vi "S4GUI_003.vi"(7 "Tab ObsEng":enum32{"Obs", "CCD modes", "Guider", "Eng"}(tab)) -> ()   [LabVIEW 2018] (continued)
                n3340 = call-dynamic "Read Interface.vi"("error in (no error)"=w7310, "Channel in"=w7313) -> ("error out"=w7327:errorcluster, "Interface.lvclass"=w7328:refnum<class "Interface.lvclass">, "Channel out"=w7345:refnum<class "Channel.lvclass">)  [unwired: 7 in]
                n3341 = call-dynamic "Write Suffix.vi"("error in (no error)"=w7327, "Suffix"=w7335, "Interface in"=w7328) -> ("error out"=w7352:errorcluster, "Interface out"=w7344:refnum<class "Interface.lvclass">)  [unwired: 7 in]
                n3342 = call-dynamic "Write ObsType.vi"("error in (no error)"=w7352, "ObsType"=w7333, "Interface in"=w7344) -> ("error out"=w7351:errorcluster, "Interface out"=w7343:refnum<class "Interface.lvclass">)  [unwired: 7 in]
                n3343 = call-dynamic "Write Object.vi"("error in (no error)"=w7351, "Object"=w7332, "Interface in"=w7343) -> ("error out"=w7350:errorcluster, "Interface out"=w7342:refnum<class "Interface.lvclass">)  [unwired: 7 in]
                n3344 = call-dynamic "Write Comments.vi"("error in (no error)"=w7350, "Comments"=w7334, "Interface in"=w7342) -> ("error out"=w7330:errorcluster, "Interface out"=w7329:refnum<class "Interface.lvclass">)  [unwired: 7 in]
                n3345 = call-dynamic "Write Observer.vi"("error in (no error)"=w7330, "Observer"=w7331, "Interface in"=w7329) -> ("error out"=w7325:errorcluster, "Interface out"=w7326:refnum<class "Interface.lvclass">)  [unwired: 7 in]
                n3346 = call-dynamic "Write Interface.vi"("error in (no error)"=w7325, "Interface.lvclass"=w7326, "Channel in"=w7345) -> ("error out"=w7321:errorcluster, "Channel out"=w7324:refnum<class "Channel.lvclass">)  [unwired: 7 in]
                n3347 = call-dynamic "Read State Machine.vi"("error in (no error)"=w7321, "Device in"=w7324) -> ("error out"=w7320:errorcluster, "State Machine.lvclass"=w7318:refnum<class "State Machine.lvclass">, "Device out"=w7323:refnum<class "Channel.lvclass">)  [unwired: 7 in]
                n3348 = call "Next State.vi"("error in (no error)"=w7320, "New_State"=12, "State Machine in"=w7318) -> ("error out"=w7319:errorcluster, "State Machine out"=w7317:refnum<class "State Machine.lvclass">)  [unwired: 7 in]
                n3349 = call-dynamic "Write State Machine.vi"("error in (no error)"=w7319, "State Machine.lvclass"=w7317, "Device in"=w7323) -> ("error out"=w7316:errorcluster, "Device out"=w7322:refnum<class "Channel.lvclass">)  [unwired: 7 in]
                n3350 = call-dynamic "Write Channel.vi"("error in (no error)"=w7316, "Channel.lvclass"=w7322, "Acquisition in"=w7340) -> ("error out"=w7338:errorcluster, "Acquisition out"=w7339:refnum<class "Acquisition.lvclass">)  [unwired: 7 in]
                n3351 = call-dynamic "Write AcquisitionA.vi"("error in (no error)"=w7338, "Acquisition.lvclass"=w7339, "S4ACS_GUI in"=w7341) -> ("error out"=w7336:errorcluster, "S4ACS_GUI out"=w7337:refnum<class "S4GUI.lvclass">)  [unwired: 7 in]
              }
              frame #1 {
                # "object"
                # "suffix"
                # "obsType"
                n3352 = call "Read AcquisitionB.vi"("error in (no error)"=w7394, "S4ACS_GUI in"=w7395) -> ("error out"=w7380:errorcluster, "Acquisition.lvclass"=w7381:refnum<class "Acquisition.lvclass">, "S4ACS_GUI out"=w7386:refnum<class "S4GUI.lvclass">)  [unwired: 7 in]
                n3353 = call-dynamic "Read Channel.vi"("error in (no error)"=w7380, "Acquisition in"=w7381) -> ("error out"=w7354:errorcluster, "Channel.lvclass"=w7356:refnum<class "Channel.lvclass">, "Acquisition out"=w7387:refnum<class "Acquisition.lvclass">)  [unwired: 7 in]
                n3354 = local read "Filter2"() -> (w7357:u8)
                n3355 = call-dynamic "Write Filter.vi"("error in (no error)"=w7354, "Filter"=w7357, "Channel in"=w7356) -> ("error out"=w7353:errorcluster, "Channel out"=w7355:refnum<class "Channel.lvclass">)  [unwired: 7 in]
                n3356 = call-dynamic "Read Interface.vi"("error in (no error)"=w7353, "Channel in"=w7355) -> ("error out"=w7368:errorcluster, "Interface.lvclass"=w7369:refnum<class "Interface.lvclass">, "Channel out"=w7382:refnum<class "Channel.lvclass">)  [unwired: 7 in]
                n3357 = call-dynamic "Write Suffix.vi"("error in (no error)"=w7368, "Suffix"=w7391, "Interface in"=w7369) -> ("error out"=w7377:errorcluster, "Interface out"=w7383:refnum<class "Interface.lvclass">)  [unwired: 7 in]
                n3358 = call-dynamic "Write ObsType.vi"("error in (no error)"=w7377, "ObsType"=w7376, "Interface in"=w7383) -> ("error out"=w7378:errorcluster, "Interface out"=w7384:refnum<class "Interface.lvclass">)  [unwired: 7 in]
                n3359 = call-dynamic "Write Object.vi"("error in (no error)"=w7378, "Object"=w7375, "Interface in"=w7384) -> ("error out"=w7379:errorcluster, "Interface out"=w7385:refnum<class "Interface.lvclass">)  [unwired: 7 in]
                n3360 = call-dynamic "Write Comments.vi"("error in (no error)"=w7379, "Comments"=w7390, "Interface in"=w7385) -> ("error out"=w7371:errorcluster, "Interface out"=w7370:refnum<class "Interface.lvclass">)  [unwired: 7 in]
                n3361 = call-dynamic "Write Observer.vi"("error in (no error)"=w7371, "Observer"=w7374, "Interface in"=w7370) -> ("error out"=w7372:errorcluster, "Interface out"=w7373:refnum<class "Interface.lvclass">)  [unwired: 7 in]
                n3362 = call-dynamic "Write Interface.vi"("error in (no error)"=w7372, "Interface.lvclass"=w7373, "Channel in"=w7382) -> ("error out"=w7361:errorcluster, "Channel out"=w7362:refnum<class "Channel.lvclass">)  [unwired: 7 in]
                n3363 = call-dynamic "Read State Machine.vi"("error in (no error)"=w7361, "Device in"=w7362) -> ("error out"=w7367:errorcluster, "State Machine.lvclass"=w7365:refnum<class "State Machine.lvclass">, "Device out"=w7360:refnum<class "Channel.lvclass">)  [unwired: 7 in]
                n3364 = call "Next State.vi"("error in (no error)"=w7367, "New_State"=12, "State Machine in"=w7365) -> ("error out"=w7366:errorcluster, "State Machine out"=w7364:refnum<class "State Machine.lvclass">)  [unwired: 7 in]
                n3365 = call-dynamic "Write State Machine.vi"("error in (no error)"=w7366, "State Machine.lvclass"=w7364, "Device in"=w7360) -> ("error out"=w7358:errorcluster, "Device out"=w7359:refnum<class "Channel.lvclass">)  [unwired: 7 in]
                n3366 = call-dynamic "Write Channel.vi"("error in (no error)"=w7358, "Channel.lvclass"=w7359, "Acquisition in"=w7387) -> ("error out"=w7389:errorcluster, "Acquisition out"=w7388:refnum<class "Acquisition.lvclass">)  [unwired: 7 in]
                n3367 = call "Write AcquisitionB.vi"("error in (no error)"=w7389, "Acquisition.lvclass"=w7388, "S4ACS_GUI in"=w7386) -> ("error out"=w7392:errorcluster, "S4ACS_GUI out"=w7393:refnum<class "S4GUI.lvclass">)  [unwired: 7 in]
              }
              frame #2 {
                # "object"
                # "suffix"
                # "obsType"
                n3368 = call-dynamic "Read AcquisitionC.vi"("error in (no error)"=w7437, "S4ACS_GUI in"=w7438) -> ("error out"=w7430:errorcluster, "Acquisition.lvclass"=w7429:refnum<class "Acquisition.lvclass">, "S4ACS_GUI out"=w7424:refnum<class "S4GUI.lvclass">)  [unwired: 7 in]
                n3369 = call-dynamic "Read Channel.vi"("error in (no error)"=w7430, "Acquisition in"=w7429) -> ("error out"=w7397:errorcluster, "Channel.lvclass"=w7399:refnum<class "Channel.lvclass">, "Acquisition out"=w7423:refnum<class "Acquisition.lvclass">)  [unwired: 7 in]
                n3370 = local read "Filter3"() -> (w7400:u8)
                n3371 = call-dynamic "Write Filter.vi"("error in (no error)"=w7397, "Filter"=w7400, "Channel in"=w7399) -> ("error out"=w7396:errorcluster, "Channel out"=w7398:refnum<class "Channel.lvclass">)  [unwired: 7 in]
                n3372 = call-dynamic "Read Interface.vi"("error in (no error)"=w7396, "Channel in"=w7398) -> ("error out"=w7415:errorcluster, "Interface.lvclass"=w7416:refnum<class "Interface.lvclass">, "Channel out"=w7428:refnum<class "Channel.lvclass">)  [unwired: 7 in]
                n3373 = call-dynamic "Write Suffix.vi"("error in (no error)"=w7415, "Suffix"=w7434, "Interface in"=w7416) -> ("error out"=w7433:errorcluster, "Interface out"=w7427:refnum<class "Interface.lvclass">)  [unwired: 7 in]
                n3374 = call-dynamic "Write ObsType.vi"("error in (no error)"=w7433, "ObsType"=w7419, "Interface in"=w7427) -> ("error out"=w7432:errorcluster, "Interface out"=w7426:refnum<class "Interface.lvclass">)  [unwired: 7 in]
                n3375 = call-dynamic "Write Object.vi"("error in (no error)"=w7432, "Object"=w7418, "Interface in"=w7426) -> ("error out"=w7431:errorcluster, "Interface out"=w7425:refnum<class "Interface.lvclass">)  [unwired: 7 in]
                n3376 = call-dynamic "Write Comments.vi"("error in (no error)"=w7431, "Comments"=w7420, "Interface in"=w7425) -> ("error out"=w7412:errorcluster, "Interface out"=w7411:refnum<class "Interface.lvclass">)  [unwired: 7 in]
                n3377 = call-dynamic "Write Observer.vi"("error in (no error)"=w7412, "Observer"=w7417, "Interface in"=w7411) -> ("error out"=w7413:errorcluster, "Interface out"=w7414:refnum<class "Interface.lvclass">)  [unwired: 7 in]
                n3378 = call-dynamic "Write Interface.vi"("error in (no error)"=w7413, "Interface.lvclass"=w7414, "Channel in"=w7428) -> ("error out"=w7406:errorcluster, "Channel out"=w7407:refnum<class "Channel.lvclass">)  [unwired: 7 in]
                n3379 = call-dynamic "Read State Machine.vi"("error in (no error)"=w7406, "Device in"=w7407) -> ("error out"=w7410:errorcluster, "State Machine.lvclass"=w7403:refnum<class "State Machine.lvclass">, "Device out"=w7405:refnum<class "Channel.lvclass">)  [unwired: 7 in]
                n3380 = call "Next State.vi"("error in (no error)"=w7410, "New_State"=12, "State Machine in"=w7403) -> ("error out"=w7409:errorcluster, "State Machine out"=w7402:refnum<class "State Machine.lvclass">)  [unwired: 7 in]
                n3381 = call-dynamic "Write State Machine.vi"("error in (no error)"=w7409, "State Machine.lvclass"=w7402, "Device in"=w7405) -> ("error out"=w7401:errorcluster, "Device out"=w7404:refnum<class "Channel.lvclass">)  [unwired: 7 in]
                n3382 = call-dynamic "Write Channel.vi"("error in (no error)"=w7401, "Channel.lvclass"=w7404, "Acquisition in"=w7423) -> ("error out"=w7421:errorcluster, "Acquisition out"=w7422:refnum<class "Acquisition.lvclass">)  [unwired: 7 in]
                n3383 = call-dynamic "Write AcquisitionC.vi"("error in (no error)"=w7421, "Acquisition.lvclass"=w7422, "S4ACS_GUI in"=w7424) -> ("error out"=w7435:errorcluster, "S4ACS_GUI out"=w7436:refnum<class "S4GUI.lvclass">)  [unwired: 7 in]
              }
              frame #3 {
                # "object"
                # "suffix"
                # "obsType"
                n3384 = call-dynamic "Read AcquisitionD.vi"("error in (no error)"=w7480, "S4ACS_GUI in"=w7481) -> ("error out"=w7473:errorcluster, "Acquisition.lvclass"=w7472:refnum<class "Acquisition.lvclass">, "S4ACS_GUI out"=w7467:refnum<class "S4GUI.lvclass">)  [unwired: 7 in]
                n3385 = call-dynamic "Read Channel.vi"("error in (no error)"=w7473, "Acquisition in"=w7472) -> ("error out"=w7440:errorcluster, "Channel.lvclass"=w7442:refnum<class "Channel.lvclass">, "Acquisition out"=w7466:refnum<class "Acquisition.lvclass">)  [unwired: 7 in]
                n3386 = local read "Filter4"() -> (w7443:u8)
                n3387 = call-dynamic "Write Filter.vi"("error in (no error)"=w7440, "Filter"=w7443, "Channel in"=w7442) -> ("error out"=w7439:errorcluster, "Channel out"=w7441:refnum<class "Channel.lvclass">)  [unwired: 7 in]
                n3388 = call-dynamic "Read Interface.vi"("error in (no error)"=w7439, "Channel in"=w7441) -> ("error out"=w7458:errorcluster, "Interface.lvclass"=w7459:refnum<class "Interface.lvclass">, "Channel out"=w7471:refnum<class "Channel.lvclass">)  [unwired: 7 in]
                n3389 = call-dynamic "Write Suffix.vi"("error in (no error)"=w7458, "Suffix"=w7477, "Interface in"=w7459) -> ("error out"=w7476:errorcluster, "Interface out"=w7470:refnum<class "Interface.lvclass">)  [unwired: 7 in]
                n3390 = call-dynamic "Write ObsType.vi"("error in (no error)"=w7476, "ObsType"=w7462, "Interface in"=w7470) -> ("error out"=w7475:errorcluster, "Interface out"=w7469:refnum<class "Interface.lvclass">)  [unwired: 7 in]
                n3391 = call-dynamic "Write Object.vi"("error in (no error)"=w7475, "Object"=w7461, "Interface in"=w7469) -> ("error out"=w7474:errorcluster, "Interface out"=w7468:refnum<class "Interface.lvclass">)  [unwired: 7 in]
                n3392 = call-dynamic "Write Comments.vi"("error in (no error)"=w7474, "Comments"=w7463, "Interface in"=w7468) -> ("error out"=w7457:errorcluster, "Interface out"=w7456:refnum<class "Interface.lvclass">)  [unwired: 7 in]
                n3393 = call-dynamic "Write Observer.vi"("error in (no error)"=w7457, "Observer"=w7460, "Interface in"=w7456) -> ("error out"=w7452:errorcluster, "Interface out"=w7451:refnum<class "Interface.lvclass">)  [unwired: 7 in]
                n3394 = call-dynamic "Write Interface.vi"("error in (no error)"=w7452, "Interface.lvclass"=w7451, "Channel in"=w7471) -> ("error out"=w7447:errorcluster, "Channel out"=w7450:refnum<class "Channel.lvclass">)  [unwired: 7 in]
                n3395 = call-dynamic "Read State Machine.vi"("error in (no error)"=w7447, "Device in"=w7450) -> ("error out"=w7455:errorcluster, "State Machine.lvclass"=w7445:refnum<class "State Machine.lvclass">, "Device out"=w7449:refnum<class "Channel.lvclass">)  [unwired: 7 in]
                n3396 = call "Next State.vi"("error in (no error)"=w7455, "New_State"=12, "State Machine in"=w7445) -> ("error out"=w7454:errorcluster, "State Machine out"=w7444:refnum<class "State Machine.lvclass">)  [unwired: 7 in]
                n3397 = call-dynamic "Write State Machine.vi"("error in (no error)"=w7454, "State Machine.lvclass"=w7444, "Device in"=w7449) -> ("error out"=w7446:errorcluster, "Device out"=w7448:refnum<class "Channel.lvclass">)  [unwired: 7 in]
                n3398 = call-dynamic "Write Channel.vi"("error in (no error)"=w7446, "Channel.lvclass"=w7448, "Acquisition in"=w7466) -> ("error out"=w7464:errorcluster, "Acquisition out"=w7465:refnum<class "Acquisition.lvclass">)  [unwired: 7 in]
                n3399 = call-dynamic "Write AcquisitionD.vi"("error in (no error)"=w7464, "Acquisition.lvclass"=w7465, "S4ACS_GUI in"=w7467) -> ("error out"=w7478:errorcluster, "S4ACS_GUI out"=w7479:refnum<class "S4GUI.lvclass">)  [unwired: 7 in]
              }
            }
          }
          frame Enabled {
          }
        }
      }
      event "object suffix", "dflat suffix", "sflat suffix", "dark suffix", "zero suffix", "focus suffix": Value Change {
        w7484 = T33 0 items=["both", "start of string", "end of string"] ("location (both)")
        # "Remove todos <\\n> e <space> do sufixo:"
        n3400 = event-data() -> ("NewVal"=w7498:string)  [unwired: 1 in, 5 out]
        n3401 = To Lower Case(string=w7498) -> (all lower case string=w7497:string)
        n3402 = call <vilib>:"Trim Whitespace.vi"("string"=w7497, "location (both)"=w7484) -> ("trimmed string"=w7496:string)
        n3403 = Search and Replace String(replace all?=TRUE ("replace all? (F)"), input string=w7496, search string="\n") -> (result string=w7495:string)  [unwired: 5 in, 3 out]
        n3404 = call <vilib>:"Space Constant.vi"() -> ("String"=w7493:string)
        n3405 = Search and Replace String(replace all?=TRUE ("replace all? (F)"), input string=w7495, search string=w7493) -> (result string=w7489:string)  [unwired: 5 in, 3 out]
        n3406 = case shown="\"DARK\"" w7490 {
          tunnel: w7489 -> [w7712 w7719 w7724 w7729 w7734 w7739]
          tunnel: w7488 -> [w7716 w7721 w7726 w7731 w7736 w7741]
          tunnel: w7487 -> [w7714 w7720 w7725 w7730 w7735 w7740]
          tunnel: [w7715 w7718 w7723 w7727 w7732 w7737] -> w7486
          tunnel: [w7713 w7717 w7722 w7728 w7733 w7738] -> w7485
          frame "OBJECT", Default {
            n3407 = local write "object suffix"(w7712) -> ()
            n3408 = call-dynamic "Write object_suffix.vi"("error in (no error)"=w7714, "object"=w7712, "S4GUI in"=w7716) -> ("error out"=w7713:errorcluster, "S4GUI out"=w7715:refnum<class "S4GUI.lvclass">)  [unwired: 7 in]
          }
          frame "DFLAT" {
            n3409 = local write "dflat suffix"(w7719) -> ()
            n3410 = call-dynamic "Write dflat_suffix.vi"("error in (no error)"=w7720, "dflat"=w7719, "S4GUI in"=w7721) -> ("error out"=w7717:errorcluster, "S4GUI out"=w7718:refnum<class "S4GUI.lvclass">)  [unwired: 7 in]
          }
          frame "SFLAT" {
            n3411 = local write "sflat suffix"(w7724) -> ()
            n3412 = call-dynamic "Write sflat_suffix.vi"("error in (no error)"=w7725, "sflat"=w7724, "S4GUI in"=w7726) -> ("error out"=w7722:errorcluster, "S4GUI out"=w7723:refnum<class "S4GUI.lvclass">)  [unwired: 7 in]
          }
          frame "DARK" {
            n3413 = local write "dark suffix"(w7729) -> ()
            n3414 = call-dynamic "Write dark_suffix.vi"("error in (no error)"=w7730, "dark"=w7729, "S4GUI in"=w7731) -> ("error out"=w7728:errorcluster, "S4GUI out"=w7727:refnum<class "S4GUI.lvclass">)  [unwired: 7 in]
          }
          frame "ZERO" {
            n3415 = local write "zero suffix"(w7734) -> ()
            n3416 = call-dynamic "Write zero_suffix.vi"("error in (no error)"=w7735, "zero"=w7734, "S4GUI in"=w7736) -> ("error out"=w7733:errorcluster, "S4GUI out"=w7732:refnum<class "S4GUI.lvclass">)  [unwired: 7 in]
          }
          frame "FOCUS" {
            n3417 = local write "focus suffix"(w7739) -> ()
            n3418 = call-dynamic "Write focus_suffix.vi"("error in (no error)"=w7740, "focus"=w7739, "S4GUI in"=w7741) -> ("error out"=w7738:errorcluster, "S4GUI out"=w7737:refnum<class "S4GUI.lvclass">)  [unwired: 7 in]
          }
        }
        n3419 = disable-structure shown="Enabled" {
          disable-tunnel: w7504 -> [w7513 _]
          disable-tunnel: w7503 -> [w7512 _]
          disable-tunnel: w7502 -> [w7511 _]
          disable-tunnel: w7501 -> [w7510 _]
          disable-tunnel: [w7509 w7711] -> w7500
          disable-tunnel: [w7508 w7710] -> w7499
          disable-tunnel: w7489 -> [w7507 _]
          disable-tunnel: w7486 -> [w7506 w7711]
          disable-tunnel: w7485 -> [w7505 w7710]
          frame Disabled {
            n3420 = stacked-sequence {
              seq-local: [w7535 _ _ _] -> [_ w7599 _ _]
              seq-local: [w7534 _ _ _] -> [_ w7598 _ _]
              seq-local: [_ w7597 _ _] -> [_ _ w7648 _]
              seq-local: [_ w7596 _ _] -> [_ _ w7647 _]
              seq-local: [_ _ w7646 _] -> [_ _ _ w7697]
              seq-local: [_ _ w7645 _] -> [_ _ _ w7696]
              tunnel: w7505 -> [w7547 _ _ _]
              tunnel: w7506 -> [w7546 _ _ _]
              tunnel: [_ _ _ w7695] -> w7509
              tunnel: [_ _ _ w7694] -> w7508
              tunnel: w7507 -> [w7533 w7595 w7644 w7693]
              tunnel: w7512 -> [w7532 w7594 w7630 w7679]
              tunnel: w7510 -> [w7531 w7580 w7629 w7678]
              tunnel: w7513 -> [w7530 w7579 w7628 w7677]
              tunnel: w7511 -> [w7529 w7578 w7627 w7676]
              frame #0 {
                # "observer"
                # "comment"
                # "object"
                # "suffix"
                # "obsType"
                n3421 = call-dynamic "Read AcquisitionA.vi"("error in (no error)"=w7547, "S4ACS_GUI in"=w7546) -> ("error out"=w7545:errorcluster, "Acquisition.lvclass"=w7544:refnum<class "Acquisition.lvclass">, "S4ACS_GUI out"=w7539:refnum<class "S4GUI.lvclass">)  [unwired: 7 in]
                n3422 = call-dynamic "Read Channel.vi"("error in (no error)"=w7545, "Acquisition in"=w7544) -> ("error out"=w7515:errorcluster, "Channel.lvclass"=w7518:refnum<class "Channel.lvclass">, "Acquisition out"=w7538:refnum<class "Acquisition.lvclass">)  [unwired: 7 in]
                n3423 = local read "Filter1"() -> (w7516:u8)
                n3424 = call-dynamic "Write Filter.vi"("error in (no error)"=w7515, "Filter"=w7516, "Channel in"=w7518) -> ("error out"=w7514:errorcluster, "Channel out"=w7517:refnum<class "Channel.lvclass">)  [unwired: 7 in]
                n3425 = call-dynamic "Read Interface.vi"("error in (no error)"=w7514, "Channel in"=w7517) -> ("error out"=w7525:errorcluster, "Interface.lvclass"=w7526:refnum<class "Interface.lvclass">, "Channel out"=w7543:refnum<class "Channel.lvclass">)  [unwired: 7 in]
                n3426 = call-dynamic "Write Suffix.vi"("error in (no error)"=w7525, "Suffix"=w7533, "Interface in"=w7526) -> ("error out"=w7550:errorcluster, "Interface out"=w7542:refnum<class "Interface.lvclass">)  [unwired: 7 in]
                n3427 = call-dynamic "Write ObsType.vi"("error in (no error)"=w7550, "ObsType"=w7531, "Interface in"=w7542) -> ("error out"=w7549:errorcluster, "Interface out"=w7541:refnum<class "Interface.lvclass">)  [unwired: 7 in]
                n3428 = call-dynamic "Write Object.vi"("error in (no error)"=w7549, "Object"=w7530, "Interface in"=w7541) -> ("error out"=w7548:errorcluster, "Interface out"=w7540:refnum<class "Interface.lvclass">)  [unwired: 7 in]
                n3429 = call-dynamic "Write Comments.vi"("error in (no error)"=w7548, "Comments"=w7532, "Interface in"=w7540) -> ("error out"=w7528:errorcluster, "Interface out"=w7527:refnum<class "Interface.lvclass">)  [unwired: 7 in]
                n3430 = call-dynamic "Write Observer.vi"("error in (no error)"=w7528, "Observer"=w7529, "Interface in"=w7527) -> ("error out"=w7523:errorcluster, "Interface out"=w7524:refnum<class "Interface.lvclass">)  [unwired: 7 in]
                n3431 = call-dynamic "Write Interface.vi"("error in (no error)"=w7523, "Interface.lvclass"=w7524, "Channel in"=w7543) -> ("error out"=w7520:errorcluster, "Channel out"=w7522:refnum<class "Channel.lvclass">)  [unwired: 7 in]
                n3432 = disable-structure shown="Enabled" {
                  disable-tunnel: w7522 -> [w7560 w7562]
                  disable-tunnel: [w7558 w7562] -> w7521
                  disable-tunnel: w7520 -> [w7557 w7561]
                  disable-tunnel: [w7552 w7561] -> w7519
                  frame Disabled {
                    n3433 = call-dynamic "Read State Machine.vi"("error in (no error)"=w7557, "Device in"=w7560) -> ("error out"=w7556:errorcluster, "State Machine.lvclass"=w7554:refnum<class "State Machine.lvclass">, "Device out"=w7559:refnum<class "Channel.lvclass">)  [unwired: 7 in]
                    n3434 = call "Next State.vi"("error in (no error)"=w7556, "New_State"=12, "State Machine in"=w7554) -> ("error out"=w7555:errorcluster, "State Machine out"=w7553:refnum<class "State Machine.lvclass">)  [unwired: 7 in]
                    n3435 = call-dynamic "Write State Machine.vi"("error in (no error)"=w7555, "State Machine.lvclass"=w7553, "Device in"=w7559) -> ("error out"=w7552:errorcluster, "Device out"=w7558:refnum<class "Channel.lvclass">)  [unwired: 7 in]
                  }
                  frame Enabled {
                  }
                }
                n3436 = call-dynamic "Write Channel.vi"("error in (no error)"=w7519, "Channel.lvclass"=w7521, "Acquisition in"=w7538) -> ("error out"=w7536:errorcluster, "Acquisition out"=w7537:refnum<class "Acquisition.lvclass">)  [unwired: 7 in]
                n3437 = call-dynamic "Write AcquisitionA.vi"("error in (no error)"=w7536, "Acquisition.lvclass"=w7537, "S4ACS_GUI in"=w7539) -> ("error out"=w7534:errorcluster, "S4ACS_GUI out"=w7535:refnum<class "S4GUI.lvclass">)  [unwired: 7 in]
              }
              frame #1 {
                # "object"
                # "suffix"
                # "obsType"
                n3438 = call "Read AcquisitionB.vi"("error in (no error)"=w7598, "S4ACS_GUI in"=w7599) -> ("error out"=w7584:errorcluster, "Acquisition.lvclass"=w7585:refnum<class "Acquisition.lvclass">, "S4ACS_GUI out"=w7590:refnum<class "S4GUI.lvclass">)  [unwired: 7 in]
                n3439 = call-dynamic "Read Channel.vi"("error in (no error)"=w7584, "Acquisition in"=w7585) -> ("error out"=w7564:errorcluster, "Channel.lvclass"=w7566:refnum<class "Channel.lvclass">, "Acquisition out"=w7591:refnum<class "Acquisition.lvclass">)  [unwired: 7 in]
                n3440 = local read "Filter2"() -> (w7567:u8)
                n3441 = call-dynamic "Write Filter.vi"("error in (no error)"=w7564, "Filter"=w7567, "Channel in"=w7566) -> ("error out"=w7563:errorcluster, "Channel out"=w7565:refnum<class "Channel.lvclass">)  [unwired: 7 in]
                n3442 = call-dynamic "Read Interface.vi"("error in (no error)"=w7563, "Channel in"=w7565) -> ("error out"=w7572:errorcluster, "Interface.lvclass"=w7573:refnum<class "Interface.lvclass">, "Channel out"=w7586:refnum<class "Channel.lvclass">)  [unwired: 7 in]
                n3443 = call-dynamic "Write Suffix.vi"("error in (no error)"=w7572, "Suffix"=w7595, "Interface in"=w7573) -> ("error out"=w7581:errorcluster, "Interface out"=w7587:refnum<class "Interface.lvclass">)  [unwired: 7 in]
                n3444 = call-dynamic "Write ObsType.vi"("error in (no error)"=w7581, "ObsType"=w7580, "Interface in"=w7587) -> ("error out"=w7582:errorcluster, "Interface out"=w7588:refnum<class "Interface.lvclass">)  [unwired: 7 in]
                n3445 = call-dynamic "Write Object.vi"("error in (no error)"=w7582, "Object"=w7579, "Interface in"=w7588) -> ("error out"=w7583:errorcluster, "Interface out"=w7589:refnum<class "Interface.lvclass">)  [unwired: 7 in]
                n3446 = call-dynamic "Write Comments.vi"("error in (no error)"=w7583, "Comments"=w7594, "Interface in"=w7589) -> ("error out"=w7575:errorcluster, "Interface out"=w7574:refnum<class "Interface.lvclass">)  [unwired: 7 in]
                n3447 = call-dynamic "Write Observer.vi"("error in (no error)"=w7575, "Observer"=w7578, "Interface in"=w7574) -> ("error out"=w7576:errorcluster, "Interface out"=w7577:refnum<class "Interface.lvclass">)  [unwired: 7 in]
                n3448 = call-dynamic "Write Interface.vi"("error in (no error)"=w7576, "Interface.lvclass"=w7577, "Channel in"=w7586) -> ("error out"=w7570:errorcluster, "Channel out"=w7571:refnum<class "Channel.lvclass">)  [unwired: 7 in]
                n3449 = disable-structure shown="Enabled" {
                  disable-tunnel: w7571 -> [w7604 w7611]
                  disable-tunnel: w7570 -> [w7603 w7610]
                  disable-tunnel: [w7601 w7611] -> w7569
                  disable-tunnel: [w7600 w7610] -> w7568
                  frame Disabled {
                    n3450 = call-dynamic "Read State Machine.vi"("error in (no error)"=w7603, "Device in"=w7604) -> ("error out"=w7609:errorcluster, "State Machine.lvclass"=w7607:refnum<class "State Machine.lvclass">, "Device out"=w7602:refnum<class "Channel.lvclass">)  [unwired: 7 in]
                    n3451 = call "Next State.vi"("error in (no error)"=w7609, "New_State"=12, "State Machine in"=w7607) -> ("error out"=w7608:errorcluster, "State Machine out"=w7606:refnum<class "State Machine.lvclass">)  [unwired: 7 in]
                    n3452 = call-dynamic "Write State Machine.vi"("error in (no error)"=w7608, "State Machine.lvclass"=w7606, "Device in"=w7602) -> ("error out"=w7600:errorcluster, "Device out"=w7601:refnum<class "Channel.lvclass">)  [unwired: 7 in]
                  }
                  frame Enabled {
                  }
                }
                n3453 = call-dynamic "Write Channel.vi"("error in (no error)"=w7568, "Channel.lvclass"=w7569, "Acquisition in"=w7591) -> ("error out"=w7593:errorcluster, "Acquisition out"=w7592:refnum<class "Acquisition.lvclass">)  [unwired: 7 in]
                n3454 = call "Write AcquisitionB.vi"("error in (no error)"=w7593, "Acquisition.lvclass"=w7592, "S4ACS_GUI in"=w7590) -> ("error out"=w7596:errorcluster, "S4ACS_GUI out"=w7597:refnum<class "S4GUI.lvclass">)  [unwired: 7 in]
              }
              frame #2 {
                # "object"
                # "suffix"
                # "obsType"
                n3455 = call-dynamic "Read AcquisitionC.vi"("error in (no error)"=w7647, "S4ACS_GUI in"=w7648) -> ("error out"=w7640:errorcluster, "Acquisition.lvclass"=w7639:refnum<class "Acquisition.lvclass">, "S4ACS_GUI out"=w7634:refnum<class "S4GUI.lvclass">)  [unwired: 7 in]
                n3456 = call-dynamic "Read Channel.vi"("error in (no error)"=w7640, "Acquisition in"=w7639) -> ("error out"=w7613:errorcluster, "Channel.lvclass"=w7615:refnum<class "Channel.lvclass">, "Acquisition out"=w7633:refnum<class "Acquisition.lvclass">)  [unwired: 7 in]
                n3457 = local read "Filter3"() -> (w7616:u8)
                n3458 = call-dynamic "Write Filter.vi"("error in (no error)"=w7613, "Filter"=w7616, "Channel in"=w7615) -> ("error out"=w7612:errorcluster, "Channel out"=w7614:refnum<class "Channel.lvclass">)  [unwired: 7 in]
                n3459 = call-dynamic "Read Interface.vi"("error in (no error)"=w7612, "Channel in"=w7614) -> ("error out"=w7625:errorcluster, "Interface.lvclass"=w7626:refnum<class "Interface.lvclass">, "Channel out"=w7638:refnum<class "Channel.lvclass">)  [unwired: 7 in]
                n3460 = call-dynamic "Write Suffix.vi"("error in (no error)"=w7625, "Suffix"=w7644, "Interface in"=w7626) -> ("error out"=w7643:errorcluster, "Interface out"=w7637:refnum<class "Interface.lvclass">)  [unwired: 7 in]
                n3461 = call-dynamic "Write ObsType.vi"("error in (no error)"=w7643, "ObsType"=w7629, "Interface in"=w7637) -> ("error out"=w7642:errorcluster, "Interface out"=w7636:refnum<class "Interface.lvclass">)  [unwired: 7 in]
                n3462 = call-dynamic "Write Object.vi"("error in (no error)"=w7642, "Object"=w7628, "Interface in"=w7636) -> ("error out"=w7641:errorcluster, "Interface out"=w7635:refnum<class "Interface.lvclass">)  [unwired: 7 in]
                n3463 = call-dynamic "Write Comments.vi"("error in (no error)"=w7641, "Comments"=w7630, "Interface in"=w7635) -> ("error out"=w7622:errorcluster, "Interface out"=w7621:refnum<class "Interface.lvclass">)  [unwired: 7 in]
                n3464 = call-dynamic "Write Observer.vi"("error in (no error)"=w7622, "Observer"=w7627, "Interface in"=w7621) -> ("error out"=w7623:errorcluster, "Interface out"=w7624:refnum<class "Interface.lvclass">)  [unwired: 7 in]
                n3465 = call-dynamic "Write Interface.vi"("error in (no error)"=w7623, "Interface.lvclass"=w7624, "Channel in"=w7638) -> ("error out"=w7619:errorcluster, "Channel out"=w7620:refnum<class "Channel.lvclass">)  [unwired: 7 in]
                n3466 = disable-structure shown="Enabled" {
                  disable-tunnel: w7620 -> [w7655 w7660]
                  disable-tunnel: w7619 -> [w7654 w7659]
                  disable-tunnel: [w7652 w7660] -> w7618
                  disable-tunnel: [w7649 w7659] -> w7617
                  frame Disabled {
                    n3467 = call-dynamic "Read State Machine.vi"("error in (no error)"=w7654, "Device in"=w7655) -> ("error out"=w7658:errorcluster, "State Machine.lvclass"=w7651:refnum<class "State Machine.lvclass">, "Device out"=w7653:refnum<class "Channel.lvclass">)  [unwired: 7 in]
                    n3468 = call "Next State.vi"("error in (no error)"=w7658, "New_State"=12, "State Machine in"=w7651) -> ("error out"=w7657:errorcluster, "State Machine out"=w7650:refnum<class "State Machine.lvclass">)  [unwired: 7 in]
                    n3469 = call-dynamic "Write State Machine.vi"("error in (no error)"=w7657, "State Machine.lvclass"=w7650, "Device in"=w7653) -> ("error out"=w7649:errorcluster, "Device out"=w7652:refnum<class "Channel.lvclass">)  [unwired: 7 in]
                  }
                  frame Enabled {
                  }
                }
                n3470 = call-dynamic "Write Channel.vi"("error in (no error)"=w7617, "Channel.lvclass"=w7618, "Acquisition in"=w7633) -> ("error out"=w7631:errorcluster, "Acquisition out"=w7632:refnum<class "Acquisition.lvclass">)  [unwired: 7 in]
                n3471 = call-dynamic "Write AcquisitionC.vi"("error in (no error)"=w7631, "Acquisition.lvclass"=w7632, "S4ACS_GUI in"=w7634) -> ("error out"=w7645:errorcluster, "S4ACS_GUI out"=w7646:refnum<class "S4GUI.lvclass">)  [unwired: 7 in]
              }
              frame #3 {
                # "object"
                # "suffix"
                # "obsType"
                n3472 = call-dynamic "Read AcquisitionD.vi"("error in (no error)"=w7696, "S4ACS_GUI in"=w7697) -> ("error out"=w7689:errorcluster, "Acquisition.lvclass"=w7688:refnum<class "Acquisition.lvclass">, "S4ACS_GUI out"=w7683:refnum<class "S4GUI.lvclass">)  [unwired: 7 in]
                n3473 = call-dynamic "Read Channel.vi"("error in (no error)"=w7689, "Acquisition in"=w7688) -> ("error out"=w7662:errorcluster, "Channel.lvclass"=w7664:refnum<class "Channel.lvclass">, "Acquisition out"=w7682:refnum<class "Acquisition.lvclass">)  [unwired: 7 in]
                n3474 = local read "Filter4"() -> (w7665:u8)
                n3475 = call-dynamic "Write Filter.vi"("error in (no error)"=w7662, "Filter"=w7665, "Channel in"=w7664) -> ("error out"=w7661:errorcluster, "Channel out"=w7663:refnum<class "Channel.lvclass">)  [unwired: 7 in]
                n3476 = call-dynamic "Read Interface.vi"("error in (no error)"=w7661, "Channel in"=w7663) -> ("error out"=w7674:errorcluster, "Interface.lvclass"=w7675:refnum<class "Interface.lvclass">, "Channel out"=w7687:refnum<class "Channel.lvclass">)  [unwired: 7 in]
                n3477 = call-dynamic "Write Suffix.vi"("error in (no error)"=w7674, "Suffix"=w7693, "Interface in"=w7675) -> ("error out"=w7692:errorcluster, "Interface out"=w7686:refnum<class "Interface.lvclass">)  [unwired: 7 in]
                n3478 = call-dynamic "Write ObsType.vi"("error in (no error)"=w7692, "ObsType"=w7678, "Interface in"=w7686) -> ("error out"=w7691:errorcluster, "Interface out"=w7685:refnum<class "Interface.lvclass">)  [unwired: 7 in]
                n3479 = call-dynamic "Write Object.vi"("error in (no error)"=w7691, "Object"=w7677, "Interface in"=w7685) -> ("error out"=w7690:errorcluster, "Interface out"=w7684:refnum<class "Interface.lvclass">)  [unwired: 7 in]
                n3480 = call-dynamic "Write Comments.vi"("error in (no error)"=w7690, "Comments"=w7679, "Interface in"=w7684) -> ("error out"=w7673:errorcluster, "Interface out"=w7672:refnum<class "Interface.lvclass">)  [unwired: 7 in]
                n3481 = call-dynamic "Write Observer.vi"("error in (no error)"=w7673, "Observer"=w7676, "Interface in"=w7672) -> ("error out"=w7671:errorcluster, "Interface out"=w7670:refnum<class "Interface.lvclass">)  [unwired: 7 in]
                n3482 = call-dynamic "Write Interface.vi"("error in (no error)"=w7671, "Interface.lvclass"=w7670, "Channel in"=w7687) -> ("error out"=w7667:errorcluster, "Channel out"=w7669:refnum<class "Channel.lvclass">)  [unwired: 7 in]
                n3483 = disable-structure shown="Enabled" {
                  disable-tunnel: w7669 -> [w7704 w7709]
                  disable-tunnel: [w7702 w7709] -> w7668
                  disable-tunnel: w7667 -> [w7701 w7708]
                  disable-tunnel: [w7700 w7708] -> w7666
                  frame Disabled {
                    n3484 = call-dynamic "Read State Machine.vi"("error in (no error)"=w7701, "Device in"=w7704) -> ("error out"=w7707:errorcluster, "State Machine.lvclass"=w7699:refnum<class "State Machine.lvclass">, "Device out"=w7703:refnum<class "Channel.lvclass">)  [unwired: 7 in]
                    n3485 = call "Next State.vi"("error in (no error)"=w7707, "New_State"=12, "State Machine in"=w7699) -> ("error out"=w7706:errorcluster, "State Machine out"=w7698:refnum<class "State Machine.lvclass">)  [unwired: 7 in]
                    n3486 = call-dynamic "Write State Machine.vi"("error in (no error)"=w7706, "State Machine.lvclass"=w7698, "Device in"=w7703) -> ("error out"=w7700:errorcluster, "Device out"=w7702:refnum<class "Channel.lvclass">)  [unwired: 7 in]
                  }
                  frame Enabled {
                  }
                }
                n3487 = call-dynamic "Write Channel.vi"("error in (no error)"=w7666, "Channel.lvclass"=w7668, "Acquisition in"=w7682) -> ("error out"=w7680:errorcluster, "Acquisition out"=w7681:refnum<class "Acquisition.lvclass">)  [unwired: 7 in]
                n3488 = call-dynamic "Write AcquisitionD.vi"("error in (no error)"=w7680, "Acquisition.lvclass"=w7681, "S4ACS_GUI in"=w7683) -> ("error out"=w7694:errorcluster, "S4ACS_GUI out"=w7695:refnum<class "S4GUI.lvclass">)  [unwired: 7 in]
              }
            }
          }
          frame Enabled {
          }
        }
      }
      event "Observer": Value Change {
        n3489 = event-data() -> ("NewVal"=w7742:string)  [unwired: 1 in, 5 out]
        n3490 = disable-structure shown="Disabled" {
          disable-tunnel: w7745 -> [w7760 w7761]
          disable-tunnel: w7742 -> [w7759 _]
          disable-tunnel: [w7758 w7761] -> w7744
          frame Disabled {
            n3491 = String Length(string=w7759) -> (length=w7757:i32)
            n3492 = Equal To 0?(x=w7757) -> (x = 0?=w7756:bool)
            n3493 = Select(t=u32 16777216, s=w7756, f=u32 16777225) -> (s? t:f=w7754:u32)
            n3494 = property on="Observer" class="Str"(error in=w7760, "Text.BGColor"=w7754) -> (error out=w7758:errorcluster)  [unwired: 1 in, 1 out]
          }
          frame Enabled {
            # "Não se usa mais o texto de fundo\ndo controle \"Observer\""
          }
        }
        n3495 = case shown="False" FALSE {
          tunnel: w7752 -> [w7770 w7968]
          tunnel: w7751 -> [w7769 _]
          tunnel: w7750 -> [w7768 _]
          tunnel: w7749 -> [w7767 _]
          tunnel: w7742 -> [w7766 _]
          tunnel: w7748 -> [w7765 _]
          tunnel: [w7764 w7968] -> w7747
          tunnel: [w7763 w7967] -> w7746
          tunnel: w7744 -> [w7762 w7967]
          frame False {
            n3496 = stacked-sequence {
              seq-local: [w7792 _ _ _] -> [_ w7856 _ _]
              seq-local: [w7791 _ _ _] -> [_ w7855 _ _]
              seq-local: [_ w7854 _ _] -> [_ _ w7905 _]
              seq-local: [_ w7853 _ _] -> [_ _ w7904 _]
              seq-local: [_ _ w7903 _] -> [_ _ _ w7954]
              seq-local: [_ _ w7902 _] -> [_ _ _ w7953]
              tunnel: w7762 -> [w7804 _ _ _]
              tunnel: w7770 -> [w7803 _ _ _]
              tunnel: [_ _ _ w7952] -> w7764
              tunnel: [_ _ _ w7951] -> w7763
              tunnel: w7768 -> [w7790 w7852 w7901 w7950]
              tunnel: w7767 -> [w7789 w7851 w7887 w7936]
              tunnel: w7765 -> [w7788 w7837 w7886 w7935]
              tunnel: w7769 -> [w7787 w7836 w7885 w7934]
              tunnel: w7766 -> [w7786 w7835 w7884 w7933]
              frame #0 {
                # "observer"
                # "comment"
                # "object"
                # "suffix"
                # "obsType"
                n3497 = call-dynamic "Read AcquisitionA.vi"("error in (no error)"=w7804, "S4ACS_GUI in"=w7803) -> ("error out"=w7802:errorcluster, "Acquisition.lvclass"=w7801:refnum<class "Acquisition.lvclass">, "S4ACS_GUI out"=w7796:refnum<class "S4GUI.lvclass">)  [unwired: 7 in]
                n3498 = call-dynamic "Read Channel.vi"("error in (no error)"=w7802, "Acquisition in"=w7801) -> ("error out"=w7772:errorcluster, "Channel.lvclass"=w7775:refnum<class "Channel.lvclass">, "Acquisition out"=w7795:refnum<class "Acquisition.lvclass">)  [unwired: 7 in]
                n3499 = local read "Filter1"() -> (w7773:u8)
                n3500 = call-dynamic "Write Filter.vi"("error in (no error)"=w7772, "Filter"=w7773, "Channel in"=w7775) -> ("error out"=w7771:errorcluster, "Channel out"=w7774:refnum<class "Channel.lvclass">)  [unwired: 7 in]
                n3501 = call-dynamic "Read Interface.vi"("error in (no error)"=w7771, "Channel in"=w7774) -> ("error out"=w7782:errorcluster, "Interface.lvclass"=w7783:refnum<class "Interface.lvclass">, "Channel out"=w7800:refnum<class "Channel.lvclass">)  [unwired: 7 in]
                n3502 = call-dynamic "Write Suffix.vi"("error in (no error)"=w7782, "Suffix"=w7790, "Interface in"=w7783) -> ("error out"=w7807:errorcluster, "Interface out"=w7799:refnum<class "Interface.lvclass">)  [unwired: 7 in]
                n3503 = call-dynamic "Write ObsType.vi"("error in (no error)"=w7807, "ObsType"=w7788, "Interface in"=w7799) -> ("error out"=w7806:errorcluster, "Interface out"=w7798:refnum<class "Interface.lvclass">)  [unwired: 7 in]
                n3504 = call-dynamic "Write Object.vi"("error in (no error)"=w7806, "Object"=w7787, "Interface in"=w7798) -> ("error out"=w7805:errorcluster, "Interface out"=w7797:refnum<class "Interface.lvclass">)  [unwired: 7 in]
                n3505 = call-dynamic "Write Comments.vi"("error in (no error)"=w7805, "Comments"=w7789, "Interface in"=w7797) -> ("error out"=w7785:errorcluster, "Interface out"=w7784:refnum<class "Interface.lvclass">)  [unwired: 7 in]
                n3506 = call-dynamic "Write Observer.vi"("error in (no error)"=w7785, "Observer"=w7786, "Interface in"=w7784) -> ("error out"=w7780:errorcluster, "Interface out"=w7781:refnum<class "Interface.lvclass">)  [unwired: 7 in]
                n3507 = call-dynamic "Write Interface.vi"("error in (no error)"=w7780, "Interface.lvclass"=w7781, "Channel in"=w7800) -> ("error out"=w7777:errorcluster, "Channel out"=w7779:refnum<class "Channel.lvclass">)  [unwired: 7 in]
                n3508 = disable-structure shown="Enabled" {
                  disable-tunnel: w7779 -> [w7817 w7819]
                  disable-tunnel: [w7815 w7819] -> w7778
                  disable-tunnel: w7777 -> [w7814 w7818]
                  disable-tunnel: [w7809 w7818] -> w7776
                  frame Disabled {
                    n3509 = call-dynamic "Read State Machine.vi"("error in (no error)"=w7814, "Device in"=w7817) -> ("error out"=w7813:errorcluster, "State Machine.lvclass"=w7811:refnum<class "State Machine.lvclass">, "Device out"=w7816:refnum<class "Channel.lvclass">)  [unwired: 7 in]
                    n3510 = call "Next State.vi"("error in (no error)"=w7813, "New_State"=12, "State Machine in"=w7811) -> ("error out"=w7812:errorcluster, "State Machine out"=w7810:refnum<class "State Machine.lvclass">)  [unwired: 7 in]
                    n3511 = call-dynamic "Write State Machine.vi"("error in (no error)"=w7812, "State Machine.lvclass"=w7810, "Device in"=w7816) -> ("error out"=w7809:errorcluster, "Device out"=w7815:refnum<class "Channel.lvclass">)  [unwired: 7 in]
                  }
                  frame Enabled {
                  }
                }
                n3512 = call-dynamic "Write Channel.vi"("error in (no error)"=w7776, "Channel.lvclass"=w7778, "Acquisition in"=w7795) -> ("error out"=w7793:errorcluster, "Acquisition out"=w7794:refnum<class "Acquisition.lvclass">)  [unwired: 7 in]
                n3513 = call-dynamic "Write AcquisitionA.vi"("error in (no error)"=w7793, "Acquisition.lvclass"=w7794, "S4ACS_GUI in"=w7796) -> ("error out"=w7791:errorcluster, "S4ACS_GUI out"=w7792:refnum<class "S4GUI.lvclass">)  [unwired: 7 in]
              }
              frame #1 {
                # "object"
                # "suffix"
                # "obsType"
                n3514 = call "Read AcquisitionB.vi"("error in (no error)"=w7855, "S4ACS_GUI in"=w7856) -> ("error out"=w7841:errorcluster, "Acquisition.lvclass"=w7842:refnum<class "Acquisition.lvclass">, "S4ACS_GUI out"=w7847:refnum<class "S4GUI.lvclass">)  [unwired: 7 in]
                n3515 = call-dynamic "Read Channel.vi"("error in (no error)"=w7841, "Acquisition in"=w7842) -> ("error out"=w7821:errorcluster, "Channel.lvclass"=w7823:refnum<class "Channel.lvclass">, "Acquisition out"=w7848:refnum<class "Acquisition.lvclass">)  [unwired: 7 in]
                n3516 = local read "Filter2"() -> (w7824:u8)
                n3517 = call-dynamic "Write Filter.vi"("error in (no error)"=w7821, "Filter"=w7824, "Channel in"=w7823) -> ("error out"=w7820:errorcluster, "Channel out"=w7822:refnum<class "Channel.lvclass">)  [unwired: 7 in]
                n3518 = call-dynamic "Read Interface.vi"("error in (no error)"=w7820, "Channel in"=w7822) -> ("error out"=w7829:errorcluster, "Interface.lvclass"=w7830:refnum<class "Interface.lvclass">, "Channel out"=w7843:refnum<class "Channel.lvclass">)  [unwired: 7 in]
                n3519 = call-dynamic "Write Suffix.vi"("error in (no error)"=w7829, "Suffix"=w7852, "Interface in"=w7830) -> ("error out"=w7838:errorcluster, "Interface out"=w7844:refnum<class "Interface.lvclass">)  [unwired: 7 in]
                n3520 = call-dynamic "Write ObsType.vi"("error in (no error)"=w7838, "ObsType"=w7837, "Interface in"=w7844) -> ("error out"=w7839:errorcluster, "Interface out"=w7845:refnum<class "Interface.lvclass">)  [unwired: 7 in]
                n3521 = call-dynamic "Write Object.vi"("error in (no error)"=w7839, "Object"=w7836, "Interface in"=w7845) -> ("error out"=w7840:errorcluster, "Interface out"=w7846:refnum<class "Interface.lvclass">)  [unwired: 7 in]
                n3522 = call-dynamic "Write Comments.vi"("error in (no error)"=w7840, "Comments"=w7851, "Interface in"=w7846) -> ("error out"=w7832:errorcluster, "Interface out"=w7831:refnum<class "Interface.lvclass">)  [unwired: 7 in]
                n3523 = call-dynamic "Write Observer.vi"("error in (no error)"=w7832, "Observer"=w7835, "Interface in"=w7831) -> ("error out"=w7833:errorcluster, "Interface out"=w7834:refnum<class "Interface.lvclass">)  [unwired: 7 in]
                n3524 = call-dynamic "Write Interface.vi"("error in (no error)"=w7833, "Interface.lvclass"=w7834, "Channel in"=w7843) -> ("error out"=w7827:errorcluster, "Channel out"=w7828:refnum<class "Channel.lvclass">)  [unwired: 7 in]
                n3525 = disable-structure shown="Enabled" {
                  disable-tunnel: w7828 -> [w7861 w7868]
                  disable-tunnel: w7827 -> [w7860 w7867]
                  disable-tunnel: [w7858 w7868] -> w7826
                  disable-tunnel: [w7857 w7867] -> w7825
                  frame Disabled {
                    n3526 = call-dynamic "Read State Machine.vi"("error in (no error)"=w7860, "Device in"=w7861) -> ("error out"=w7866:errorcluster, "State Machine.lvclass"=w7864:refnum<class "State Machine.lvclass">, "Device out"=w7859:refnum<class "Channel.lvclass">)  [unwired: 7 in]
                    n3527 = call "Next State.vi"("error in (no error)"=w7866, "New_State"=12, "State Machine in"=w7864) -> ("error out"=w7865:errorcluster, "State Machine out"=w7863:refnum<class "State Machine.lvclass">)  [unwired: 7 in]
                    n3528 = call-dynamic "Write State Machine.vi"("error in (no error)"=w7865, "State Machine.lvclass"=w7863, "Device in"=w7859) -> ("error out"=w7857:errorcluster, "Device out"=w7858:refnum<class "Channel.lvclass">)  [unwired: 7 in]
                  }
                  frame Enabled {
                  }
                }
                n3529 = call-dynamic "Write Channel.vi"("error in (no error)"=w7825, "Channel.lvclass"=w7826, "Acquisition in"=w7848) -> ("error out"=w7850:errorcluster, "Acquisition out"=w7849:refnum<class "Acquisition.lvclass">)  [unwired: 7 in]
                n3530 = call "Write AcquisitionB.vi"("error in (no error)"=w7850, "Acquisition.lvclass"=w7849, "S4ACS_GUI in"=w7847) -> ("error out"=w7853:errorcluster, "S4ACS_GUI out"=w7854:refnum<class "S4GUI.lvclass">)  [unwired: 7 in]
              }
              frame #2 {
                # "object"
                # "suffix"
                # "obsType"
                n3531 = call-dynamic "Read AcquisitionC.vi"("error in (no error)"=w7904, "S4ACS_GUI in"=w7905) -> ("error out"=w7897:errorcluster, "Acquisition.lvclass"=w7896:refnum<class "Acquisition.lvclass">, "S4ACS_GUI out"=w7891:refnum<class "S4GUI.lvclass">)  [unwired: 7 in]
                n3532 = call-dynamic "Read Channel.vi"("error in (no error)"=w7897, "Acquisition in"=w7896) -> ("error out"=w7870:errorcluster, "Channel.lvclass"=w7872:refnum<class "Channel.lvclass">, "Acquisition out"=w7890:refnum<class "Acquisition.lvclass">)  [unwired: 7 in]
                n3533 = local read "Filter3"() -> (w7873:u8)
                n3534 = call-dynamic "Write Filter.vi"("error in (no error)"=w7870, "Filter"=w7873, "Channel in"=w7872) -> ("error out"=w7869:errorcluster, "Channel out"=w7871:refnum<class "Channel.lvclass">)  [unwired: 7 in]
                n3535 = call-dynamic "Read Interface.vi"("error in (no error)"=w7869, "Channel in"=w7871) -> ("error out"=w7882:errorcluster, "Interface.lvclass"=w7883:refnum<class "Interface.lvclass">, "Channel out"=w7895:refnum<class "Channel.lvclass">)  [unwired: 7 in]
                n3536 = call-dynamic "Write Suffix.vi"("error in (no error)"=w7882, "Suffix"=w7901, "Interface in"=w7883) -> ("error out"=w7900:errorcluster, "Interface out"=w7894:refnum<class "Interface.lvclass">)  [unwired: 7 in]
                n3537 = call-dynamic "Write ObsType.vi"("error in (no error)"=w7900, "ObsType"=w7886, "Interface in"=w7894) -> ("error out"=w7899:errorcluster, "Interface out"=w7893:refnum<class "Interface.lvclass">)  [unwired: 7 in]
                n3538 = call-dynamic "Write Object.vi"("error in (no error)"=w7899, "Object"=w7885, "Interface in"=w7893) -> ("error out"=w7898:errorcluster, "Interface out"=w7892:refnum<class "Interface.lvclass">)  [unwired: 7 in]
                n3539 = call-dynamic "Write Comments.vi"("error in (no error)"=w7898, "Comments"=w7887, "Interface in"=w7892) -> ("error out"=w7879:errorcluster, "Interface out"=w7878:refnum<class "Interface.lvclass">)  [unwired: 7 in]
                n3540 = call-dynamic "Write Observer.vi"("error in (no error)"=w7879, "Observer"=w7884, "Interface in"=w7878) -> ("error out"=w7880:errorcluster, "Interface out"=w7881:refnum<class "Interface.lvclass">)  [unwired: 7 in]
                n3541 = call-dynamic "Write Interface.vi"("error in (no error)"=w7880, "Interface.lvclass"=w7881, "Channel in"=w7895) -> ("error out"=w7876:errorcluster, "Channel out"=w7877:refnum<class "Channel.lvclass">)  [unwired: 7 in]
                n3542 = disable-structure shown="Enabled" {
                  disable-tunnel: w7877 -> [w7912 w7917]
                  disable-tunnel: w7876 -> [w7911 w7916]
                  disable-tunnel: [w7909 w7917] -> w7875
                  disable-tunnel: [w7906 w7916] -> w7874
                  frame Disabled {
                    n3543 = call-dynamic "Read State Machine.vi"("error in (no error)"=w7911, "Device in"=w7912) -> ("error out"=w7915:errorcluster, "State Machine.lvclass"=w7908:refnum<class "State Machine.lvclass">, "Device out"=w7910:refnum<class "Channel.lvclass">)  [unwired: 7 in]
                    n3544 = call "Next State.vi"("error in (no error)"=w7915, "New_State"=12, "State Machine in"=w7908) -> ("error out"=w7914:errorcluster, "State Machine out"=w7907:refnum<class "State Machine.lvclass">)  [unwired: 7 in]
                    n3545 = call-dynamic "Write State Machine.vi"("error in (no error)"=w7914, "State Machine.lvclass"=w7907, "Device in"=w7910) -> ("error out"=w7906:errorcluster, "Device out"=w7909:refnum<class "Channel.lvclass">)  [unwired: 7 in]
                  }
                  frame Enabled {
                  }
                }
                n3546 = call-dynamic "Write Channel.vi"("error in (no error)"=w7874, "Channel.lvclass"=w7875, "Acquisition in"=w7890) -> ("error out"=w7888:errorcluster, "Acquisition out"=w7889:refnum<class "Acquisition.lvclass">)  [unwired: 7 in]
                n3547 = call-dynamic "Write AcquisitionC.vi"("error in (no error)"=w7888, "Acquisition.lvclass"=w7889, "S4ACS_GUI in"=w7891) -> ("error out"=w7902:errorcluster, "S4ACS_GUI out"=w7903:refnum<class "S4GUI.lvclass">)  [unwired: 7 in]
              }
              frame #3 {
                # "object"
                # "suffix"
                # "obsType"
                n3548 = call-dynamic "Read AcquisitionD.vi"("error in (no error)"=w7953, "S4ACS_GUI in"=w7954) -> ("error out"=w7946:errorcluster, "Acquisition.lvclass"=w7945:refnum<class "Acquisition.lvclass">, "S4ACS_GUI out"=w7940:refnum<class "S4GUI.lvclass">)  [unwired: 7 in]
                n3549 = call-dynamic "Read Channel.vi"("error in (no error)"=w7946, "Acquisition in"=w7945) -> ("error out"=w7919:errorcluster, "Channel.lvclass"=w7921:refnum<class "Channel.lvclass">, "Acquisition out"=w7939:refnum<class "Acquisition.lvclass">)  [unwired: 7 in]
                n3550 = local read "Filter4"() -> (w7922:u8)
                n3551 = call-dynamic "Write Filter.vi"("error in (no error)"=w7919, "Filter"=w7922, "Channel in"=w7921) -> ("error out"=w7918:errorcluster, "Channel out"=w7920:refnum<class "Channel.lvclass">)  [unwired: 7 in]
